vi "Get factors.vi"(8 "error in (no error)":errorcluster, 11 "x":i32) -> (0 "error out":errorcluster, 1 "T = x is a perfect square":bool, 2 "T = x is prime":bool, 3 "Factors out":T1[](array[typedef]), 4 "T = x is a perfect cube":bool, 6 "Execution time (ms)":u32)   [LabVIEW 2021, in "Numeric Utilities.lvlib"]
uses:
  Numeric Utilities.lvlib
  Factors cluster.ctl
  Named Timers/Named Timers.lvlib
panel:
  out "Dev: Factors-inside loop":T1[](array[typedef])
  in  "Dev: Stop Button":bool
  out "Loop iteration":i32
  # "Development\ncontrols/indicators useful for development and testing, but which are not outputs of the VI"
  # "Input\nInputs to the VI"
  # "Output\nOutputs of the VI"
  # "Description\n\nBlank VI with error handling case. \n\nSummarize the use of this VI in this space."
  # "2^31 -1 is prime. The largest number that can be stored in a 32-bit signed integer is prime."
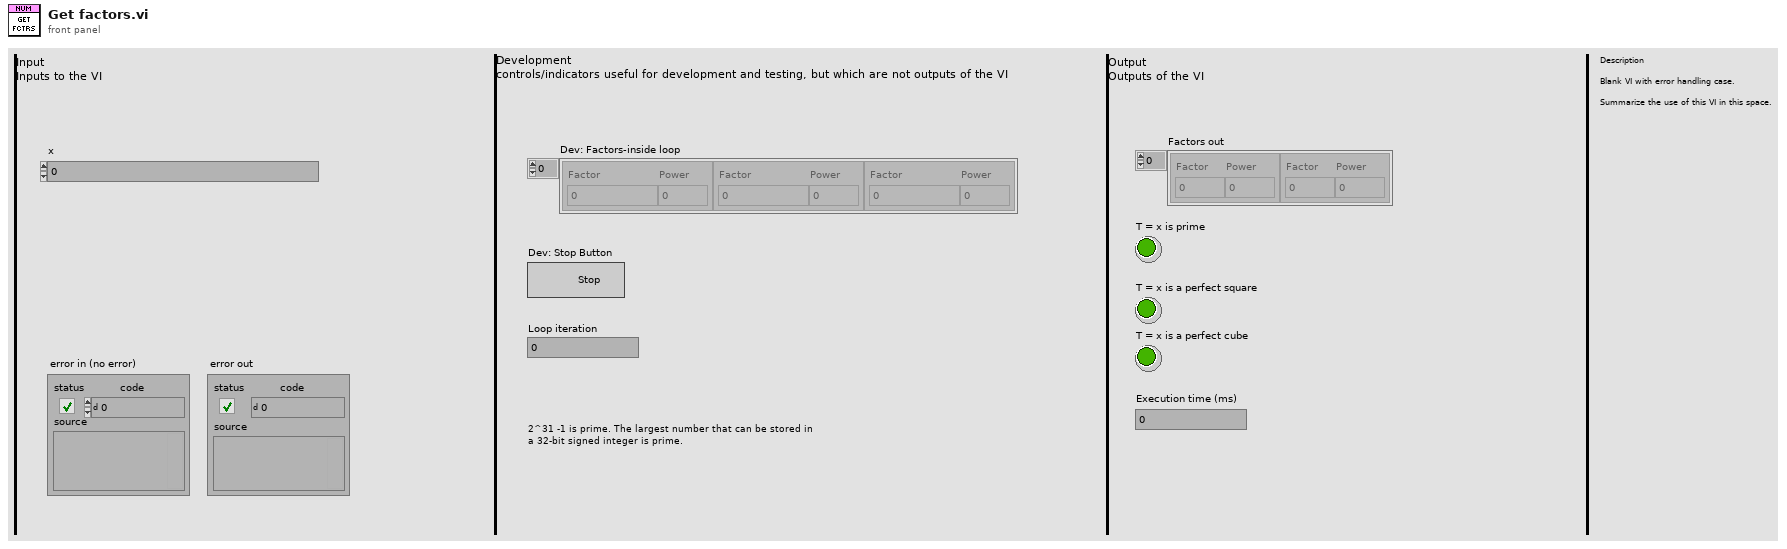
[diagram p1: front panel]
types:
  T1 = typedef "Numeric Utilities.lvlib/Factors cluster.ctl" = cluster{"Factor":i32, "Power":i32}
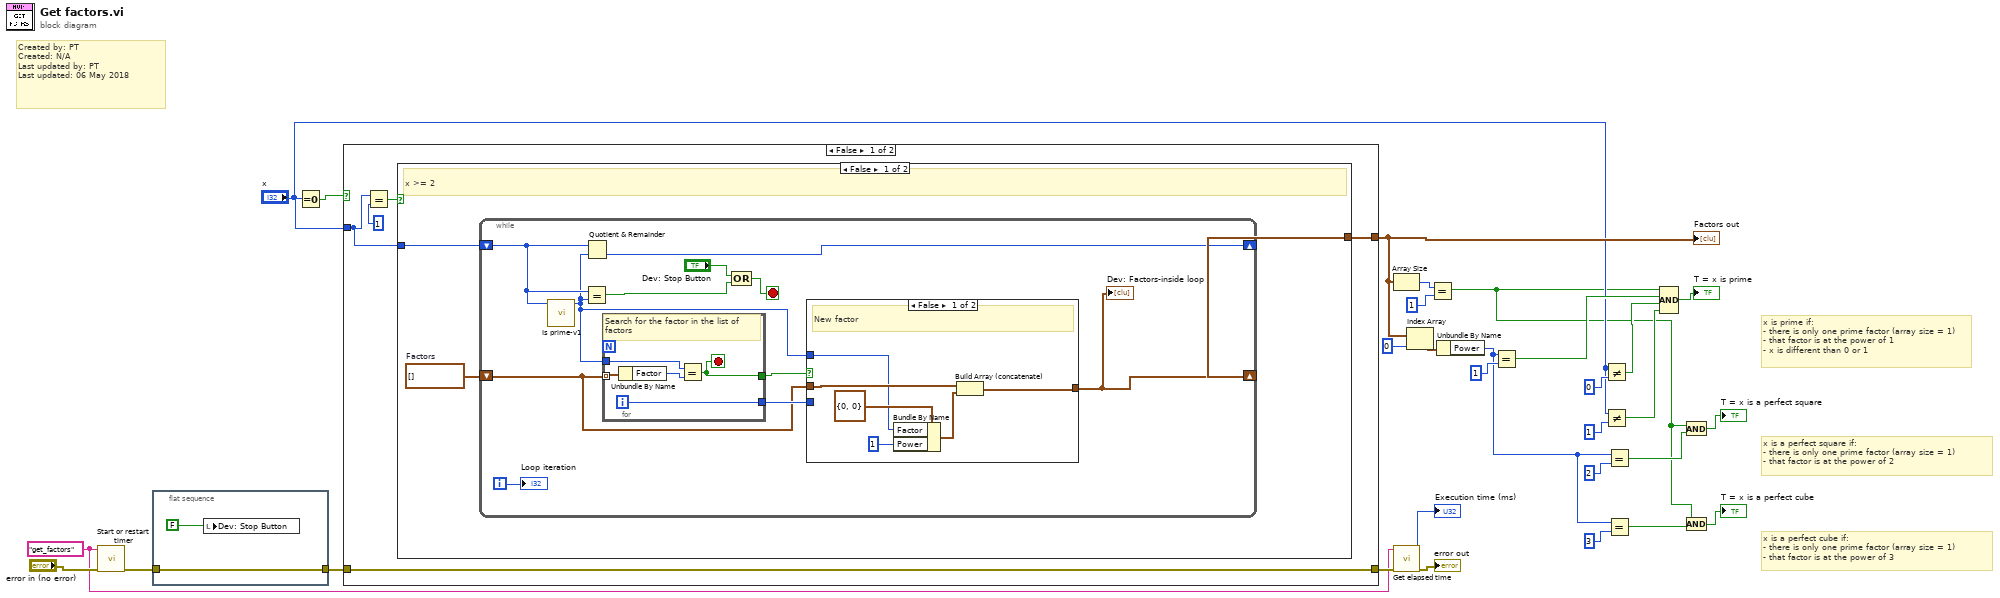
[diagram p0: block diagram]
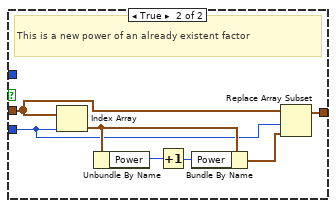
[diagram p2: hidden frame]
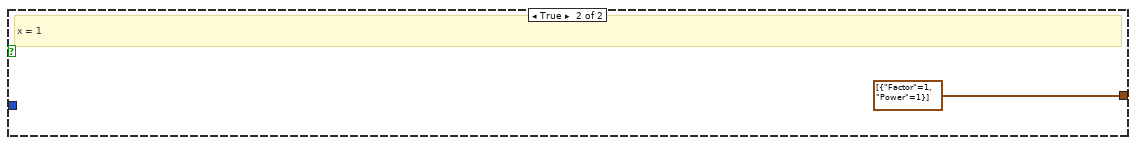
[diagram p3: hidden frame]
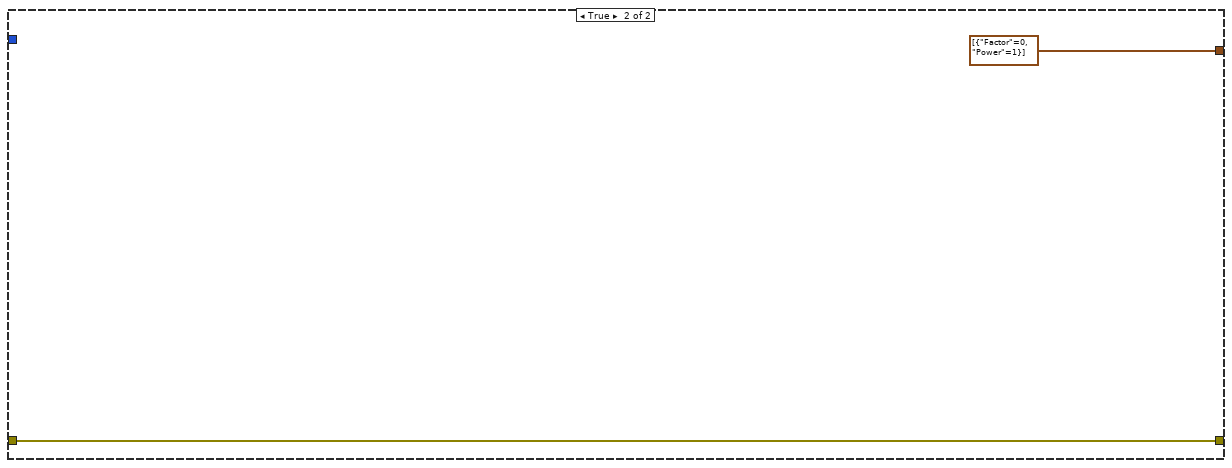
[diagram p4: hidden frame]
diagram:
  w25 = "get_factors" ("Timer name")
  # "x is a perfect cube if:\n- there is only one prime factor (array size = 1)\n- that factor is at the power of 3"
  # "x is a perfect square if:\n- there is only one prime factor (array size = 1)\n- that factor is at the power of 2"
  # "Created by: PT\nCreated: N/A\nLast updated by: PT\nLast updated: 06 May 2018"
  # "x is prime if:\n- there is only one prime factor (array size = 1)\n- that factor is at the power of 1\n- x is different than 0 or 1"
  n1 = call "Start or restart timer.vi"("error in (no error)"="error in (no error)", "Timer name"=w25) -> ("error out"=w2:errorcluster)  [unwired: 9 in]
  n2 = flat-sequence {
    tunnel: w2 -> [w30]
    tunnel: [w30] -> w1
    frame #0 {
      n3 = local write "Dev: Stop Button"(FALSE ("Stop Button")) -> ()
    }
  }
  n4 = Equal To 0?(x="x") -> (x = 0?=w29:bool)
  n5 = case shown="False" w29 {
    tunnel: [w36 T1[] [{"Factor"=0, "Power"=1}]] -> w21
    tunnel: "x" -> [w34 _]
    tunnel: w1 -> [w35 w71]
    tunnel: [w35 w71] -> w26
    frame False {
      n6 = Equal?(x=w34, y=1) -> (x = y?=w32:bool)
      n7 = case shown="False" w32 {
        tunnel: [w37 T1[] [{"Factor"=1, "Power"=1}]] -> w36
        tunnel: w34 -> [w39 _]
        frame False {
          w38 = T1[] []  # Factors
          # "x >= 2"
          n8 = while {
            shift-right: [w49] -> _
            shift-left: w39 -> [w50]
            shift-right: [w40] -> w37
            shift-left: w38 -> [w46]
            i -> [w44]
            stop <- w42 stop-if-true
            n9 = call "Is prime-v1.vi"("x"=w50) -> ("First factor"=w45:i32)  [unwired: 8 in, 2 out]
            n10 = Equal?(x=w50, y=w45) -> (x = y?=w43:bool)
            n11 = Quotient & Remainder(x=w50, y=w45) -> (floor(x/y)=w49:i32)  [unwired: 1 out]
            n12 = for {
              tunnel: w46 -> [w68] mode=indexing
              tunnel: w45 -> [w66]
              tunnel: [w65] -> w48
              tunnel: [w64] -> w47
              i -> [w64]
              stop <- w65 stop-if-true
              # "Search for the factor in the list of factors"
              n13 = Unbundle By Name(w68) -> ("Factor"=w67:i32)
              n14 = Equal?(x=w66, y=w67) -> (x = y?=w65:bool)
            }
            n15 = Compound Arithmetic op=OR("Dev: Stop Button", w43) -> (w42:bool)
            n16 = case shown="False" w48 {
              tunnel: w47 -> [_ w58]
              tunnel: w46 -> [w56 w63]
              tunnel: [w51 w57] -> w40
              tunnel: w45 -> [w54 _]
              frame False {
                # "New factor"
                n17 = Bundle By Name(cluster=T1 {"Factor"=0, "Power"=0} ("Factors cluster"), "Factor"=w54, "Power"=1) -> (w52:T1)
                n18 = Build Array (concatenate)(w56, w52) -> (w51:T1[])
              }
              frame True {
                # "This is a new power of an already existent factor"
                n19 = Index Array(array=w63, index=w58) -> (element=w62:T1)
                n20 = Unbundle By Name(w62) -> ("Power"=w60:i32)
                n21 = Increment(x=w60) -> (x+1=w61:i32)
                n22 = Bundle By Name(cluster=w62, "Power"=w61) -> (w59:T1)
                n23 = Replace Array Subset(array=w63, new element=w59, index=w58) -> (w57:T1[])
              }
            }
            "Dev: Factors-inside loop" <- w40
            "Loop iteration" <- w44
          }
        }
        frame True {
          # "x = 1"
        }
      }
    }
    frame True {
    }
  }
  "Factors out" <- w21
  n24 = Array Size(array=w21) -> (size(s)=w23:i32)
  n25 = call "Get elapsed time.vi"("error in (no error)"=w26, "Timer name"=w25) -> ("error out"=→"error out":errorcluster, "Elapsed time (ms)"=→"Execution time (ms)":u32)  [unwired: 6 in, 2 out]
  n26 = Index Array(array=w21, index=0) -> (element=w19:T1)
  n27 = Equal?(x=w23, y=1) -> (x = y?=w4:bool)
  n28 = Unbundle By Name(w19) -> ("Power"=w3:i32)
  n29 = Equal?(x=w3, y=1) -> (x = y?=w17:bool)
  n30 = Not Equal?(x="x", y=0) -> (x != y?=w14:bool)
  n31 = Not Equal?(x="x", y=1) -> (x != y?=w12:bool)
  n32 = Equal?(x=w3, y=2) -> (x = y?=w8:bool)
  n33 = Equal?(x=w3, y=3) -> (x = y?=w5:bool)
  n34 = Compound Arithmetic op=AND(w4, w17, w14, w12) -> (→"T = x is prime":bool)
  n35 = Compound Arithmetic op=AND(w4, w8) -> (→"T = x is a perfect square":bool)
  n36 = Compound Arithmetic op=AND(w4, w5) -> (→"T = x is a perfect cube":bool)
